vi "VI Server_Get Text Ring Item Names.vi"(7 "Label":string, 8 "error in":errorcluster, 9 "Single Instance (T)":bool=TRUE, 11 "VI Server Cluster":T1) -> (0 "error out":errorcluster, 1 "Control Reference":refnum<vi>, 2 "Strings []":string[](array[string]), 3 "VI Server Custer.DUP":T1={"Labels"=["Label", "Size", "Font", "Heght", "Width", "Ledding Denominator", "Ledding Nominator", "Label Number", "Microstep Resolution", "X", "Y", "Z", "Italic?", "Underlined?"], "Refs"=[], "VI Ref"=refnum}, 4 "Value":u16, 6 "Label.Text":string)   [LabVIEW 2020, in "VI Server Toolkit LV2013.lvlib"]
doc: "Returns item names (STR array) of the Text Ring."
uses:
  VI Server Toolkit LV2013.lvlib
  VI Server_TypeDefs/VI Server_RefsCluster.ctl
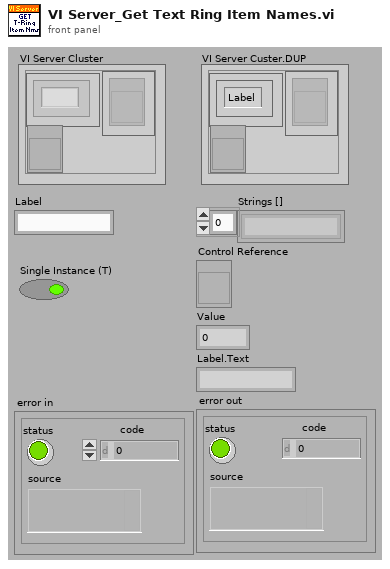
[diagram p1: front panel]
types:
  T1 = typedef "VI Server_RefsCluster.ctl" = cluster{"Labels":string[], "Refs":refnum<vi>[], "VI Ref":refnum<vi>}
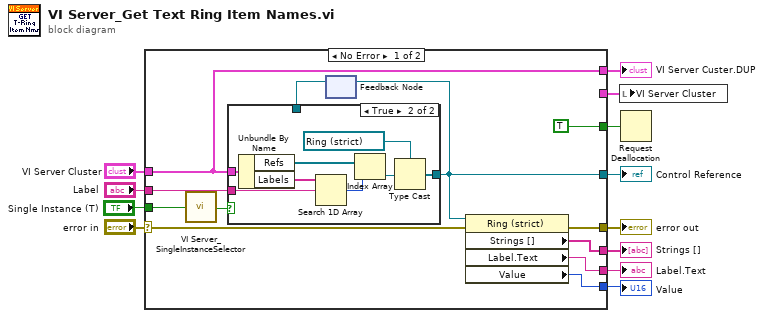
[diagram p0: block diagram]
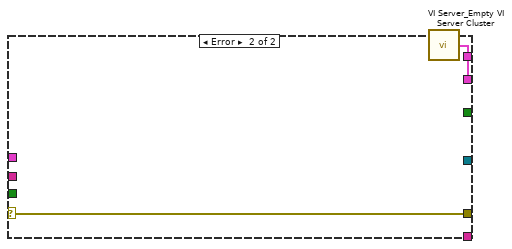
[diagram p3: hidden frame]
diagram:
  n1 = case shown="No Error" "error in" {
    selector: "error in" -> [w23 w35]
    tunnel: "Label" -> [w24 _]
    tunnel: "VI Server Cluster" -> [w20 _]
    tunnel: [w22 w35] -> w12
    tunnel: [w14 _] -> w8
    tunnel: [w21 _] -> w7
    tunnel: [w20 _] -> w6
    tunnel: [w19 _] -> w5
    tunnel: [w18 _] -> w4
    tunnel: [TRUE _] -> w3
    tunnel: [_ w34] -> w2
    tunnel: "Single Instance (T)" -> [w15 _]
    frame No Error {
      n2 = call "VI Server_SingleInstanceSelector.vi"("Single Instance (T)"=w15) -> ("Single Instance.OUT"=w16:bool)  [unwired: 6 in]
      n3 = feedback #1() -> (w13:refnum<vi>)  [unwired: 1 in]
      n4 = case shown="True" w16 {
        tunnel: w24 -> [_ w32]
        tunnel: [w25 w27] -> w14
        tunnel: w20 -> [_ w26]
        tunnel: w13 -> [w25 _]
        frame False {
        }
        frame True {
          n5 = Unbundle By Name(w26) -> ("Refs"=w30:refnum<vi>[], "Labels"=w33:string[])
          n6 = Search 1D Array(1D array=w33, element=w32) -> (index of element=w31:i32)  [unwired: 1 out]
          n7 = Index Array(array=w30, index=w31) -> (element=w29:refnum<vi>)
          n8 = Type Cast(type=refnum<vi> refnum ("Ring"), x=w29) -> (*(type *) &x=w27:refnum<vi>)
        }
      }
      n9 = feedback-in #1(w14) -> ()
      n10 = property class="Ring (strict)"(reference=w14, error in=w23) -> (error out=w22:errorcluster, "Strings []"=w19:string[], "Label.Text"=w21:string, "Value"=w18:u16)  [unwired: 1 out]
    }
    frame Error {
      n11 = call "VI Server_Empty VI Server Cluster.vi"() -> ("VI Server Cluster"=w34:T1)  [unwired: 7 in]
    }
  }
  "error out" <- w12
  "VI Server Custer.DUP" <- w6
  "Control Reference" <- w8
  "Label.Text" <- w7
  "Strings []" <- w5
  "Value" <- w4
  n12 = local write "VI Server Cluster"(w2) -> ()
  n13 = Request Deallocation(w3) -> ()
